vi "Setup Channel.vi"   [LabVIEW 2020, in "Actor Pub Sub Channels.lvlib"]
uses:
  Actor Pub Sub Channels.lvlib
  Pub Sub Message Channel/Pub Sub Message Channel.lvclass
  Pub Sub Retaining Message Channel/Pub Sub Retaining Message Channel.lvclass
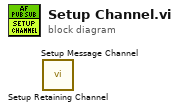
[diagram p0: block diagram]
diagram:
  n1 = call "Setup Retaining Channel.vi"() -> ()  [unwired: 10 in, 2 out]
  n2 = call "Setup Message Channel.vi"() -> ()  [unwired: 10 in, 2 out]
